vi "Control and acquisition.vi"() -> ()   [LabVIEW 2017]
uses:
  <vilib>/vision/Image Controls.llb/IMAQ Image.ctl
  <vilib>/vision/driver/IMAQdx.llb/IMAQdx Buffer Number Mode.ctl
  <vilib>/Utility/error.llb/DialogType.ctl
  <vilib>/vision/driver/IMAQdx.llb/IMAQdx Acquisition Mode.ctl
  <vilib>/DAQmx/write.llb/DAQmx Write (Analog 1D DBL NChan 1Samp).vi
  <vilib>/DAQmx/write.llb/DAQmx Write (Analog 1D Wfm NChan NSamp).vi
  <vilib>/DAQmx/create/channels.llb/DAQmx Create Channel (CO-Pulse Generation-Time).vi
  <vilib>/DAQmx/configure/timing.llb/DAQmx Timing (Implicit).vi
  <vilib>/vision/driver/Vision Acquisition Express Utility VIs.llb/Vision Acquisition Path Convert (Path).vi
  <vilib>/DAQmx/create/channels.llb/DAQmx Create Channel (AO-Voltage-Basic).vi
  <vilib>/DAQmx/miscellaneous.llb/DAQmx Fill In Error Info.vi
  <vilib>/DAQmx/configure/timing.llb/DAQmx Timing (Use Waveform).vi
  <vilib>/DAQmx/configure/trigger.llb/DAQmx Start Trigger (Digital Edge).vi
  <vilib>/vision/driver/NI_Vision_Acquisition_Software.lvlib
  <resource>/objmgr/imaqdx.rc
  <resource>/objmgr/daqmx.rc
  <vilib>/vision/NI_Vision_Development_Module.lvlib
panel:
  in  "?":dbl=40.0 format="%.1f"
  in  "Center laser\nfor power\nmeasurements":bool
  in  "Duration (ms)":dbl=10.5
  out "Multipoint":bool
  out "How to use:":string
  in  "Select mode:":u16(ring) items=["Line stimulation", "Hexagon shape stimulation"]
  out "FAST number of buffers":u32
  out "WIDE number of buffers":u32
  in  "?":dbl=2.0 format="%#_2f"
  in  "?":u32=500
  in  "?":dbl=2.0 format="%.1f"
  in  "Jump size (cm)":dbl=0.03791
  out "XY Graph":cluster{dbl[], dbl[]}(graph)
  out "(M)ULTI":bool
  in  "timeout (s)":dbl=10.0 format="%0.2f"
  in  "stop (T)":bool=TRUE
  in  "error in":errorcluster
  out "error out 2":errorcluster caption="error out"
  out "task out":refnum<k21>
  out "Time of previous recording":timestamp
  out "Trigger camera":bool
  in  "Initial Delay (ms)":dbl=0.5 caption="Initial delay (s)" format="%#.1f"
  in  "Pulse duration":dbl=0.003 caption="Pulse duration (ms)" format="%#.1p"
  in  "Number of pulses":i32=10
  in  "Interpulse interval":dbl=0.097 format="%#.1p"
  out "Boolean":bool
  out "LostBufferCount":u32
  out "new picture":picture
  in  "error in 3":errorcluster caption="error in"
  out "Image Out 2":T1(plugin-control)
  out "All Image Buffers Out 2":T1[](array[typedef])
  out "error out 3":errorcluster
  in  "Stop (F) 2":bool caption="Stop (F)"
  out "?":dbl format="%1_2f"
  out "Recording 2":bool
  out "Wide":bool
  in  "error in 2":errorcluster caption="error in"
  out "All Image Buffers Out":T1[](array[typedef])
  out "error out":errorcluster
  in  "Stop (F)":bool
  out "Frame Rate":dbl
  out "BufferCount":u32
  out "Recording":bool
  out "Fast":bool
  in  "color(black)":u32(colorbox)=6618880
  out "Xsaved1":dbl format="%#_2g"
  out "Ysaved1":dbl format="%#_2g"
  out "Ysaved2":dbl format="%#_2g"
  out "Xsaved2":dbl format="%#_2g"
  out "'1'":bool
  out "'2'":bool
  out "X":dbl format="%#_3f"
  out "Y":dbl format="%#_3f"
  out "Image Out":T1(plugin-control)
  out "x .and. y?":bool
  # "Cameras"
  # "Wide"
  # "Fast"
  # "FPS"
  # "Length (s)"
  # "Re-run VI to change these settings"
  # "Pulse generator"
  # "Re-run VI to change these settings"
  # "Patterned stimulation \nmode"
  # "Monitoring"
  # "System ready?"
  # "Stimulation shape:"
  # "Cameras?"
  # "Galvos?"
  # "Laser?"
  # "ON"
  # "FPS"
  # "FPS"
  # "rec?"
  # "rec?"
  # "Patterns?"
  # "ON"
types:
  T1 = typedef "IMAQ Image.ctl" = refnum<image>
  T2 = cluster{"Width":u16, "Style":enum32{"Solid", "Dash", "Dot", "DashDot", "DashDotDot"}}
  T3 = typedef "LVPoint32TypeDef.ctl" = cluster{"Horizontal":i32, "Vertical":i32}
  T4 = typedef "DialogType.ctl" = u16
  T5 = typedef "NI_Vision_Acquisition_Software.lvlib/IMAQdx Buffer Number Mode.ctl" = enum32{"Next", "Last", "Buffer Number", "Every", "Last New"}
  T6 = typedef "NI_Vision_Acquisition_Software.lvlib/IMAQdx Acquisition Mode.ctl" = enum32{"One Shot", "Continuous"}
  T7 = typedef "IMAQdx.ctl" = refnum<k21>
  T8 = cluster{"File Type":string, "Quality":u32, "Compress":bool, "Lossless":bool, "Ratio":sgl, "Codec":string, "Frame Rate":u32, "Limit Frames":bool, "FAST number of buffers":u32}
  T9 = cluster{"File Type":string, "Quality":u32, "Compress":bool, "Lossless":bool, "Ratio":sgl, "Codec":string, "Frame Rate":u32, "Limit Frames":bool, "WIDE number of buffers":u32}
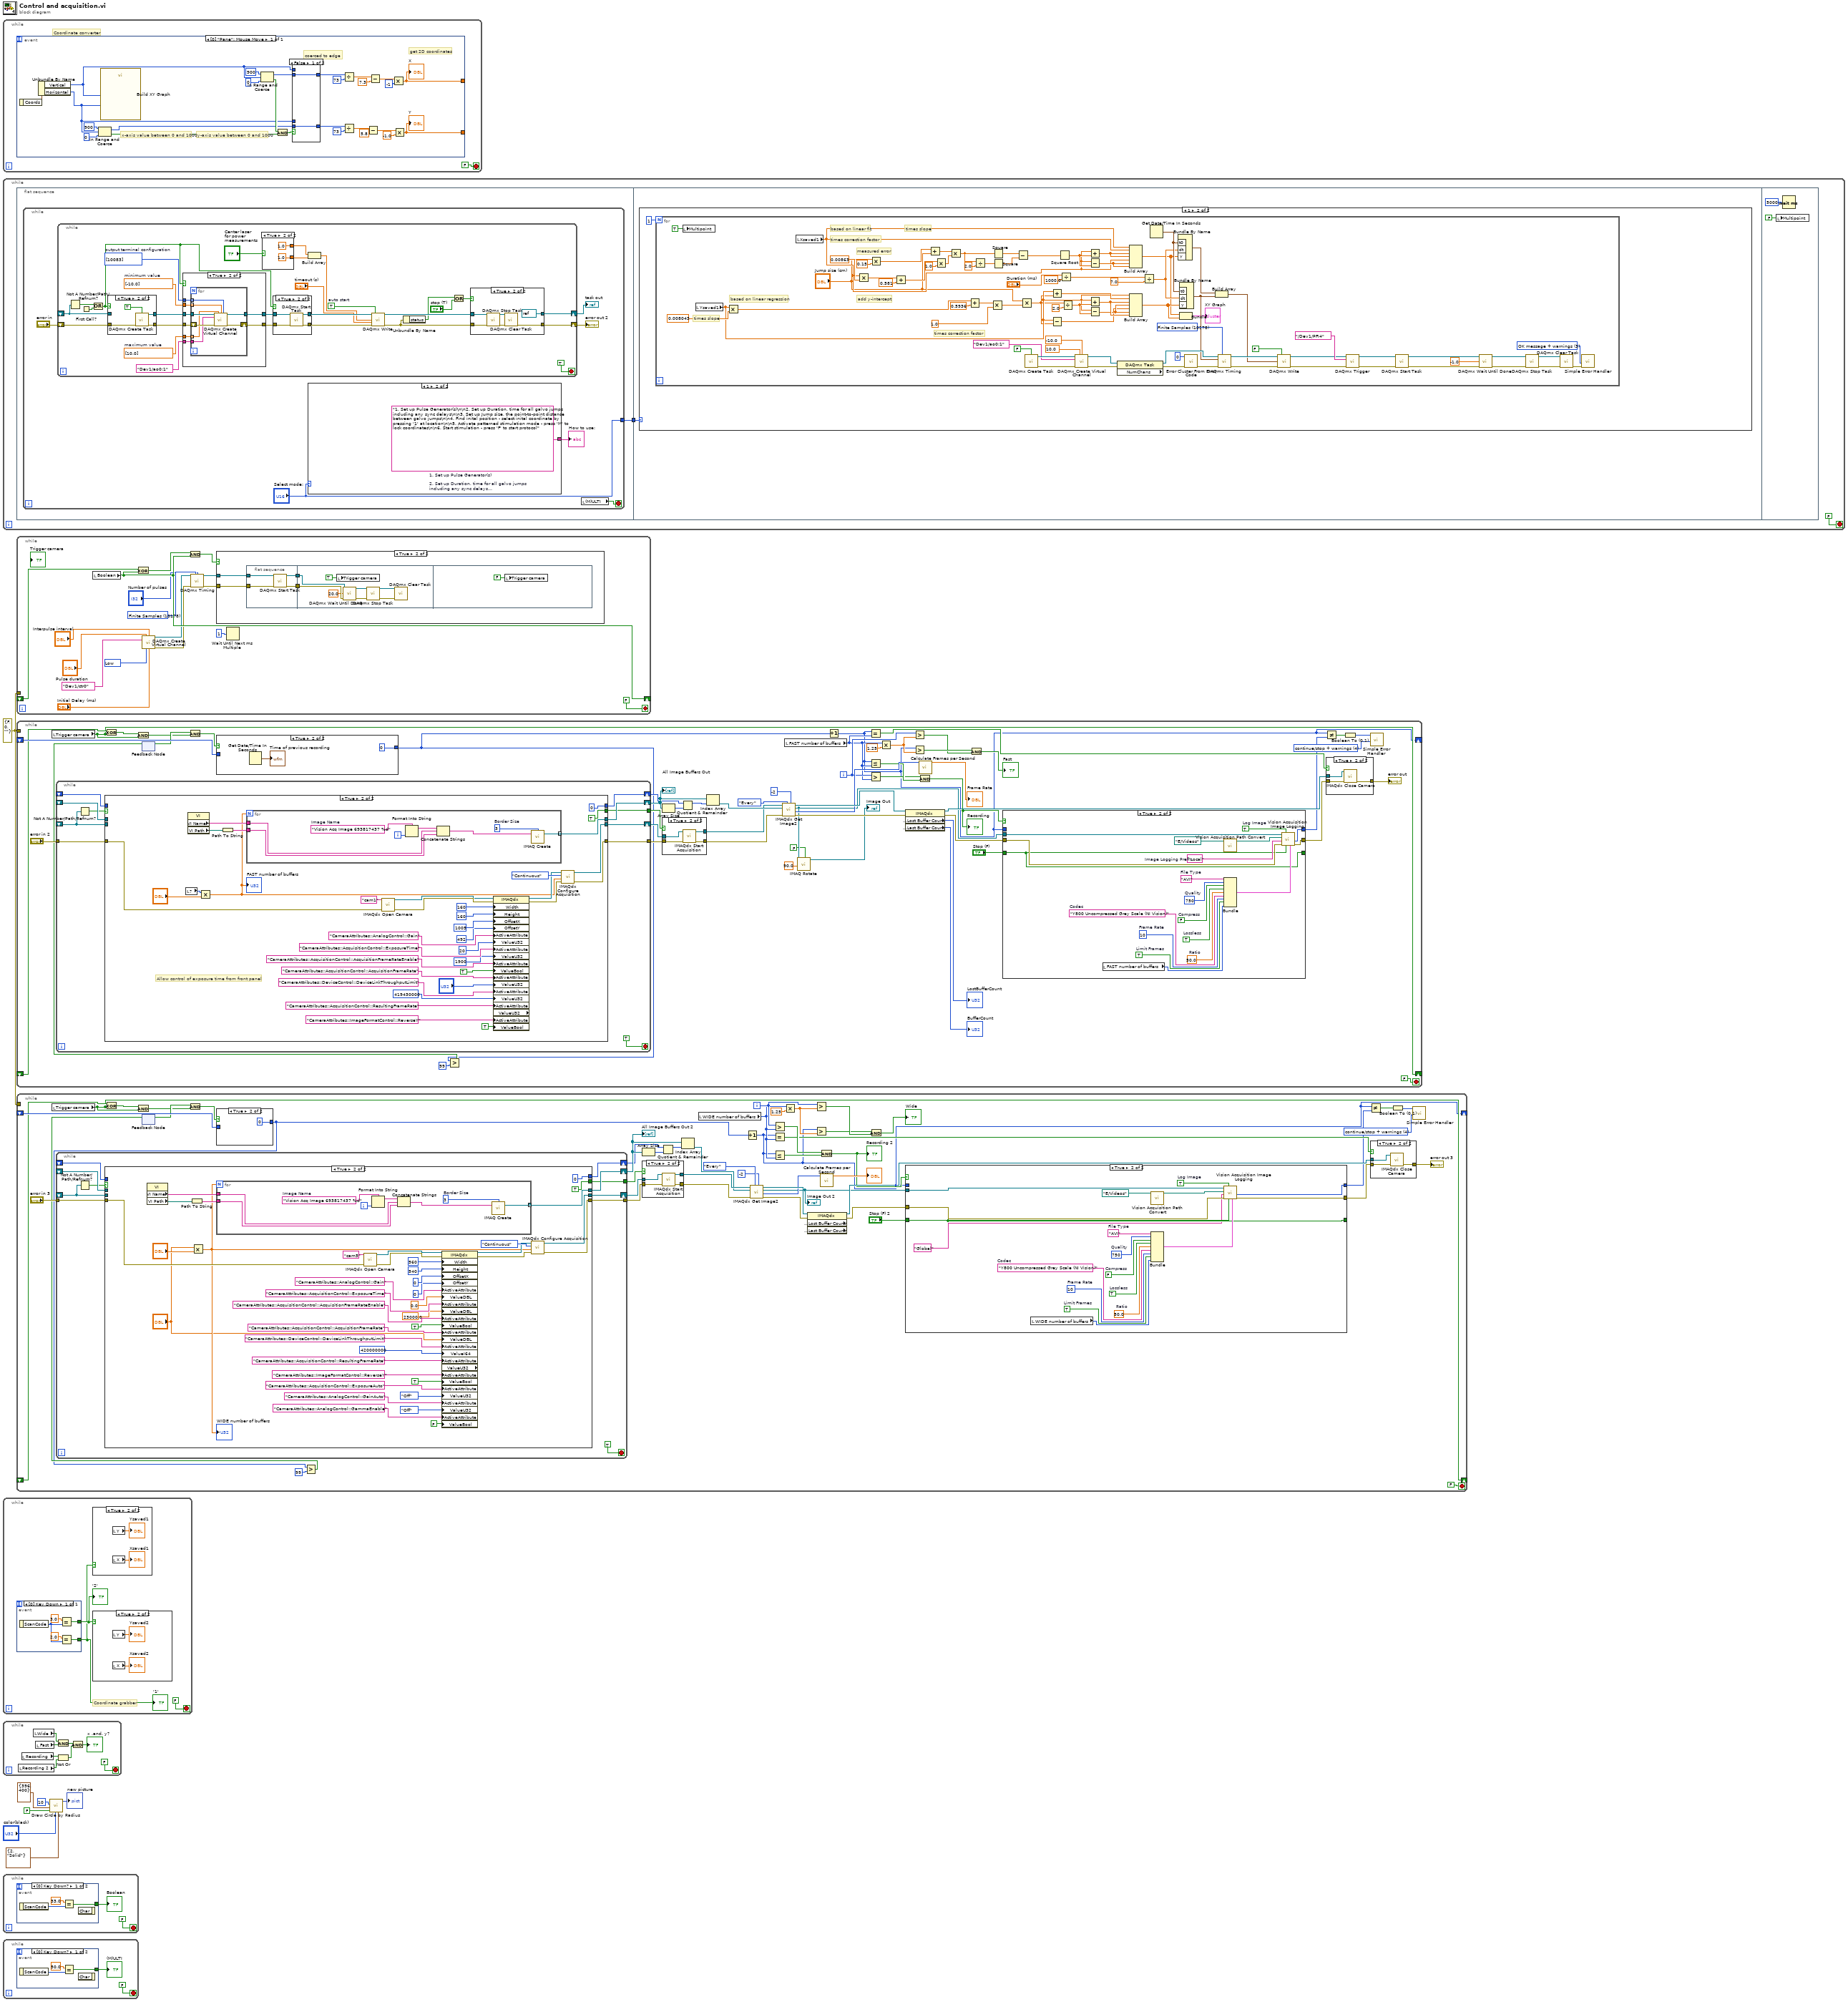
[diagram p0: block diagram]
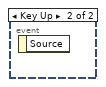
[diagram p2: hidden frame]
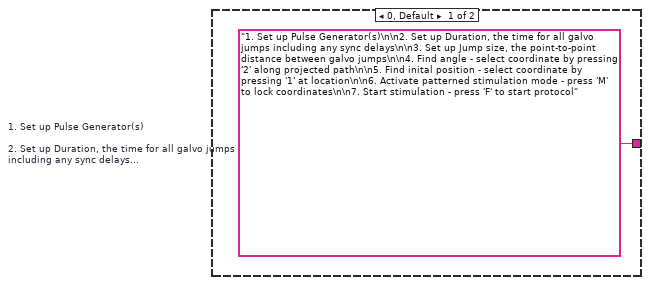
[diagram p3: hidden frame]
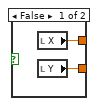
[diagram p4: hidden frame]
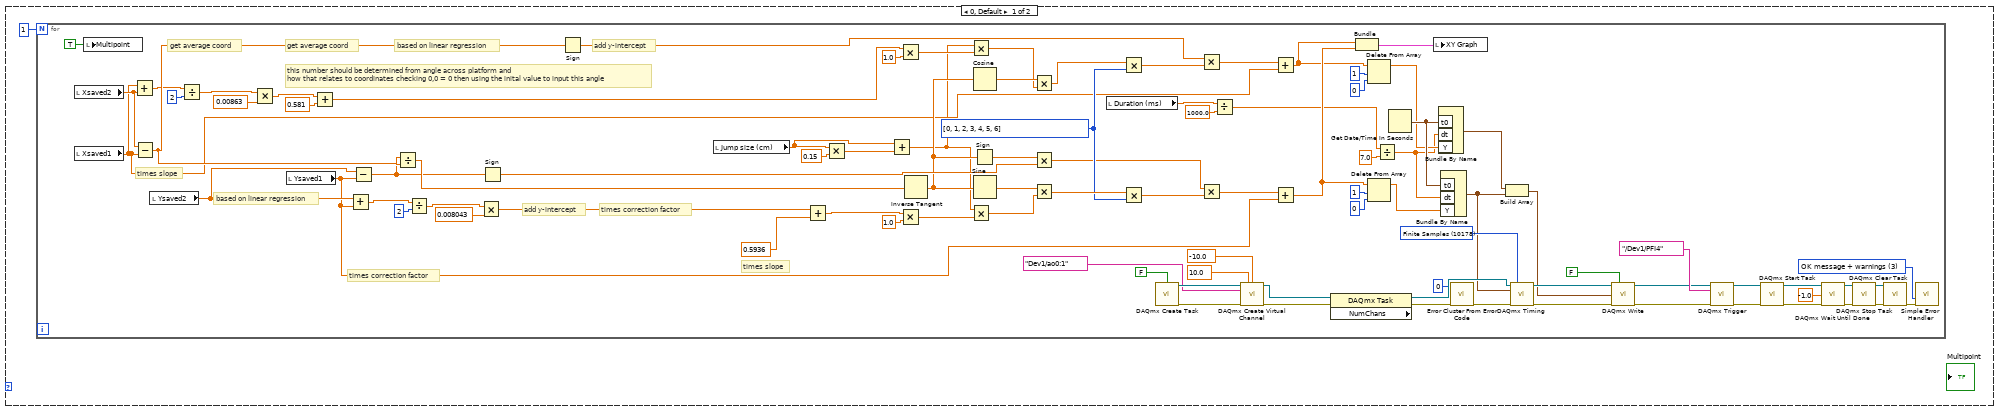
[diagram p9: hidden frame]
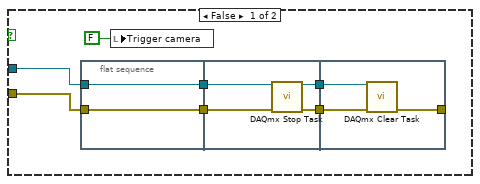
[diagram p10: hidden frame]
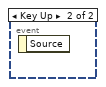
[diagram p11: hidden frame]
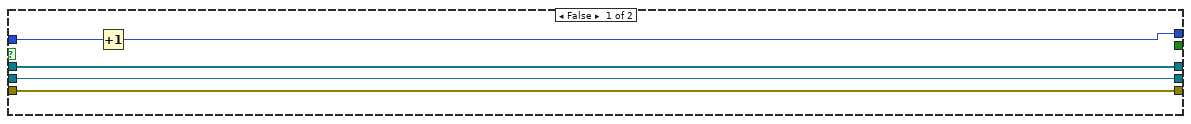
[diagram p16: hidden frame]
diagram:
  w1 = errorcluster {"status"=FALSE, "code"=0, "source"=""} ("error constant")
  n1 = while {
    stop <- FALSE ("stop") stop-if-true
    # "Coordinate converter"
    n2 = event shown="[0] \"Pane\": Mouse Move" {
      selector: _ -> [_]
      dyn-events: _ -> [_]
      timeout: _ -> [_]
      tunnel: [w14] -> _
      tunnel: [w12] -> _
      event Mouse Move {
        # "coerced to edge"
        # "y-axis value between 0 and 1000"
        # "x-axis value between 0 and 1000"
        # "get 2D coordinates"
        n3 = event-data() -> ("Coords"=w15:T3)  [unwired: 1 in]
        n4 = Unbundle By Name(w15) -> ("Vertical"=w10:i32, "Horizontal"=w9:i32)
        n5 = In Range and Coerce(upper limit=900, x=w9, lower limit=0) -> (coerced(x)=w22:i32, In Range?=w30:bool)
        n6 = call "Build XY Graph"("Y Input"=w9, "X Input"=w10) -> ()  [unwired: 8 in, 2 out]
        n7 = In Range and Coerce(upper limit=900, x=w10, lower limit=0) -> (coerced(x)=w23:i32, In Range?=w29:bool)
        n8 = And(x=w29, y=w30) -> (x .and. y?=w26:bool)
        n9 = case shown="False" w26 {
          tunnel: [w36 w38] -> w25
          tunnel: w10 -> [_ w38]
          tunnel: w9 -> [_ w37]
          tunnel: [w35 w37] -> w24
          tunnel: w23 -> [w36 _]
          tunnel: w22 -> [w35 _]
          frame False {
          }
          frame True {
          }
        }
        n10 = Divide(x=w25, y=73) -> (x/y=w17:dbl)
        n11 = Divide(x=w24, y=73) -> (x/y=w19:dbl)
        n12 = Subtract(x=w19, y=5.8) -> (x-y=w13:dbl)
        n13 = Subtract(x=w17, y=7.3) -> (x-y=w16:dbl)
        n14 = Multiply(x=w16, y=-1) -> (x*y=w14:dbl)
        "X" <- w14
        n15 = Multiply(x=w13, y=-1.0) -> (x*y=w12:dbl)
        "Y" <- w12
      }
    }
  }
  n16 = while {
    stop <- FALSE stop-if-true
    n17 = flat-sequence {
      tunnel: [w41] -> w39
      tunnel: w39 -> [w121]
      frame #0 {
        n18 = while {
          tunnel: ["Select mode:"] -> w41
          stop <- w44 stop-if-true
          n19 = while {
            shift-right: [w61] -> w45
            shift-left: _ -> [w75]
            shift-right: [w59] -> w46
            shift-left: "error in" -> [w76]
            stop <- TRUE stop-if-true
            w63 = TRUE  # auto start
            w69 = i32[] [10083] items=["Default"=-1, "RSE"=10083, "Differential"=10106, "Pseudodifferential"=12529]  # output terminal configuration
            w70 = dbl[] [10.0]  # maximum value
            w71 = dbl[] [-10.0]  # minimum value
            n20 = Not A Number/Path/Refnum?(number/path/refnum=w75) -> (NaN/Path/Refnum?=w74:bool)
            n21 = First Call?() -> (First Call?: T/F=w77:bool)
            n22 = Or(x=w74, y=w77) -> (x .or. y?=w68:bool)
            n23 = case shown="True" w68 {
              tunnel: [w116 w120] -> w73
              tunnel: w75 -> [w116 _]
              tunnel: [w115 w119] -> w72
              tunnel: w76 -> [w115 w117]
              frame False {
              }
              frame True {
                n24 = call <vilib>:"DAQmx Create Task.vi"("auto cleanup"=TRUE, "error in"=w117) -> ("task out"=w120:refnum<k21>, "error out"=w119:errorcluster)  [unwired: 12 in]
              }
            }
            n25 = case shown="True" w68 {
              tunnel: [w98 w104] -> w67
              tunnel: w73 -> [w98 w106]
              tunnel: [w97 w103] -> w66
              tunnel: w72 -> [w97 w105]
              tunnel: w71 -> [_ w102]
              tunnel: w70 -> [_ w101]
              tunnel: w69 -> [_ w100]
              tunnel: tag "Dev1/ao0:1" ("Physical Channel") -> [_ w99]
              frame False {
              }
              frame True {
                n26 = for {
                  tunnel: w106 -> [w114]
                  tunnel: [w112] -> w104
                  tunnel: w102 -> [w110] mode=indexing
                  tunnel: w101 -> [w109] mode=indexing
                  shift-right: [w111] -> w103
                  shift-left: w105 -> [w113]
                  tunnel: w100 -> [w108] mode=indexing
                  tunnel: w99 -> [w107]
                  n27 = call-poly <vilib>:"DAQmx Create Virtual Channel.vi"("task in"=w114, "maximum value"=w109, "minimum value"=w110, "output terminal configuration"=w108, "physical channels"=w107, "error in"=w113) -> ("task out"=w112:refnum<k21>, "error out"=w111:errorcluster)  [unwired: 8 in]
                }
              }
            }
            n28 = case shown="True" "Center laser\nfor power\nmeasurements" {
              tunnel: [w80 1.0 ("X")] -> w52
              tunnel: [w79 1.0 ("Y")] -> w51
              frame False {
                n29 = local read "X"() -> (w80:dbl)
                n30 = local read "Y"() -> (w79:dbl)
              }
              frame True {
              }
            }
            n31 = case shown="True" w68 {
              tunnel: [w92 w95] -> w65
              tunnel: w67 -> [w92 w96]
              tunnel: [w91 w93] -> w64
              tunnel: w66 -> [w91 w94]
              frame False {
              }
              frame True {
                n32 = call <vilib>:"DAQmx Start Task.vi"("task/channels in"=w96, "error in"=w94) -> ("task out"=w95:refnum<k21>, "error out"=w93:errorcluster)  [unwired: 12 in]
              }
            }
            n33 = Build Array(w52, w51) -> (w53:dbl[])
            n34 = call-poly <vilib>:"DAQmx Write.vi"("task/channels in"=w65, "auto start"=w63, "data"=w53, "timeout"="timeout (s)", "error in"=w64) -> ("task out"=w60:refnum<k21>, "error out"=w58:errorcluster)  [unwired: 8 in, 1 out]
            n35 = Unbundle By Name(w58) -> ("status"=w57:bool)
            n36 = Or(x=w57, y="stop (T)") -> (x .or. y?=w55:bool)
            n37 = case shown="True" w55 {
              tunnel: [w84 refnum<k21> refnum ("task in")] -> w61
              tunnel: w60 -> [w84 w90]
              tunnel: [w83 w87] -> w59
              tunnel: w58 -> [w83 w89]
              frame False {
              }
              frame True {
                n38 = call <vilib>:"DAQmx Stop Task.vi"("task/channels in"=w90, "error in"=w89) -> ("task out"=w86:refnum<k21>, "error out"=w88:errorcluster)  [unwired: 12 in]
                n39 = call <vilib>:"DAQmx Clear Task.vi"("task in"=w86, "error in"=w88) -> ("error out"=w87:errorcluster)  [unwired: 13 in]
              }
            }
          }
          "error out 2" <- w46
          "task out" <- w45
          n40 = case shown="1" "Select mode:" {
            tunnel: [w48 w49] -> w43
            frame 0, Default {
              w48 = "1. Set up Pulse Generator(s)\n\n2. Set up Duration, the time for all galvo jumps including any sync delays\n\n3. Set up Jump size, the point-to-point distance between galvo jumps\n\n4. Find angle - select coordinate by pressing '2' along projected path\n\n5. Find inital position - select coordinate by pressing '1' at location\n\n6. Activate patterned stimulation mode - press 'M' to lock coordinates\n\n7. Start stimulation - press 'F' to start protocol"  # 1. Set up Pulse Generator(s)  2. Set up Duration, the time for all galvo jumps including any sync delays  3. Set up Jump size, the point-to-point distance between galvo jumps  4. Find angle - select coordinate by pressing '2' along projected path  5. Find inital position - select coordinate by pressing '1' at location  6. Activate patterned stimulation mode - press 'M' to lock coordinates  7. Start stimulation - press 'F' to start protocol
            }
            frame 1 {
              w49 = "1. Set up Pulse Generator(s)\n\n2. Set up Duration, time for all galvo jumps including any sync delays\n\n3. Set up Jump size, the point-to-point distance between galvo jumps\n\n4. Find inital position - select inital coordinate by pressing '1' at location\n\n5. Activate patterned stimulation mode - press 'M' to lock coordinates\n\n6. Start stimulation - press 'F' to start protocol"  # 1. Set up Pulse Generator(s)  2. Set up Duration, time for all galvo jumps including any sync delays  3. Set up Jump size, the point-to-point distance between galvo jumps  4. Find inital position - select inital coordinate by pressing '1' at location  5. Activate patterned stimulation mode - press 'M' to lock coordinates  6. Start stimulation - press 'F' to start protocol
            }
          }
          "How to use:" <- w43
          n41 = local read "(M)ULTI"() -> (w44:bool)
        }
      }
      frame #1 {
        n42 = case shown="1" w121 {
          frame 0, Default {
            n43 = for {
              N: 1 -> [_]
              w154 = i32[] [0, 1, 2, 3, 4, 5, 6]
              w200 = 10178 items=["Finite Samples"=10178, "Continuous Samples"=10123] ("sample mode")
              w210 = T4 3 items=["no dialog", "OK message", "continue or stop message", "OK message + warnings", "continue/stop + warnings"] ("type of dialog (OK msg:1)")
              # "times correction factor"
              # "add y-intercept"
              # "times slope"
              # "get average coord"
              # "based on linear regression"
              # "times correction factor"
              # "add y-intercept"
              # "times slope"
              # "get average coord"
              # "based on linear regression"
              # "this number should be determined from angle across platform and \nhow that relates to coordinates checking 0,0 = 0 then using the inital value to input this angle"
              n44 = local read "Xsaved2"() -> (w161:dbl)
              n45 = local read "Xsaved1"() -> (w132:dbl)
              n46 = local write "Multipoint"(TRUE ("Multipoint")) -> ()
              n47 = Add(x=w132, y=w161) -> (x+y=w179:dbl)
              n48 = Subtract(x=w161, y=w132) -> (x-y=w184:dbl)
              n49 = local read "Ysaved2"() -> (w160:dbl)
              n50 = Divide(x=w179, y=2) -> (x/y=w177:dbl)
              n51 = Multiply(x=w177, y=0.00863) -> (x*y=w175:dbl)
              n52 = local read "Ysaved1"() -> (w142:dbl)
              n53 = Add(x=w175, y=0.581) -> (x+y=w173:dbl)
              n54 = Add(x=w160, y=w142) -> (x+y=w170:dbl)
              n55 = Subtract(x=w160, y=w142) -> (x-y=w183:dbl)
              n56 = Divide(x=w183, y=w184) -> (x/y=w190:dbl)
              n57 = Divide(x=w170, y=2) -> (x/y=w168:dbl)
              n58 = Multiply(x=w168, y=0.008043) -> (x*y=w166:dbl)
              n59 = Sign(1:w183) -> (0:w140:dbl)
              n60 = Sign(1:w184) -> (0:w143:dbl)
              n61 = local read "Jump size (cm)"() -> (w129:dbl)
              n62 = Add(x=w166, y=0.5936) -> (x+y=w164:dbl)
              n63 = Multiply(x=w129, y=0.15) -> (x*y=w130:dbl)
              n64 = Add(x=w129, y=w130) -> (x+y=w123:dbl)
              n65 = Multiply(x=w173, y=1.0) -> (x*y=w171:dbl)
              n66 = Multiply(x=w164, y=1.0) -> (x*y=w162:dbl)
              n67 = Inverse Tangent(1:w190) -> (0:w139:dbl)
              n68 = Multiply(x=w123, y=w171) -> (x*y=w138:dbl)
              n69 = Multiply(x=w123, y=w162) -> (x*y=w141:dbl)
              n70 = Cosine(x=w139) -> (cos(x)=w157:dbl)
              n71 = Sign(1:w139) -> (0:w149:dbl)
              n72 = Sine(x=w139) -> (sin(x)=w155:dbl)
              n73 = Multiply(x=w157, y=w138) -> (x*y=w158:dbl)
              n74 = Multiply(x=w149, y=w140) -> (x*y=w148:dbl)
              n75 = Multiply(x=w155, y=w141) -> (x*y=w156:dbl)
              n76 = local read "Duration (ms)"() -> (w133:dbl)
              n77 = Multiply(x=w158, y=w154) -> (x*y=w150:dbl[])
              n78 = Multiply(x=w156, y=w154) -> (x*y=w152:dbl[])
              n79 = call <vilib>:"DAQmx Create Task.vi"("auto cleanup"=FALSE) -> ("task out"=w203:refnum<k21>, "error out"=w204:errorcluster)  [unwired: 13 in]
              n80 = Multiply(x=w143, y=w150) -> (x*y=w151:dbl[])
              n81 = Multiply(x=w148, y=w152) -> (x*y=w153:dbl[])
              n82 = Divide(x=w133, y=1000.0) -> (x/y=w126:dbl)
              n83 = call-poly <vilib>:"DAQmx Create Virtual Channel.vi"("task in"=w203, "maximum value"=10.0 ("Maximum Value"), "minimum value"=-10.0 ("Minimum Value"), "physical channels"=tag "Dev1/ao0:1" ("Physical Channel"), "error in"=w204) -> ("task out"=w214:refnum<k21>, "error out"=w212:errorcluster)  [unwired: 9 in]
              n84 = Add(x=w151, y=w132) -> (x+y=w134:dbl[])
              n85 = Add(x=w153, y=w142) -> (x+y=w135:dbl[])
              n86 = property class="DAQmx Task" props=["NumChans"](reference=w214, error in=w212) -> (reference out=w206:refnum<k21>, error out=w213:errorcluster)  [unwired: 1 out]
              n87 = Bundle(w134, w135) -> (w159:cluster{dbl[], dbl[]})  [unwired: 1 in]
              n88 = Delete From Array(array=w134, length=1, index=0) -> (array with subset deleted=w136:dbl[])  [unwired: 1 out]
              n89 = Delete From Array(array=w135, length=1, index=0) -> (array with subset deleted=w137:dbl[])  [unwired: 1 out]
              n90 = Divide(x=w126, y=7.0) -> (x/y=w124:dbl)
              n91 = Get Date/Time In Seconds() -> (seconds since 1Jan1904=w199:timestamp)
              n92 = local write "XY Graph"(w159) -> ()
              n93 = Bundle By Name("t0"=w199, "dt"=w124, "Y"=w136) -> (w181:waveform(dbl))  [unwired: 1 in]
              n94 = Bundle By Name("t0"=w199, "dt"=w124, "Y"=w137) -> (w180:waveform(dbl))  [unwired: 1 in]
              n95 = call <vilib>:"Error Cluster From Error Code.vi"("error in (no error)"=w213, "error code (0)"=0) -> ("error out"=w197:errorcluster)  [unwired: 7 in]
              n96 = Build Array(w181, w180) -> (w189:waveform(dbl)[])
              n97 = call-poly <vilib>:"DAQmx Timing.vi"("task/channels in"=w206, "sample mode"=w200, "waveform"=w180, "error in"=w197) -> ("task out"=w202:refnum<k21>, "error out"=w198:errorcluster)  [unwired: 10 in]
              n98 = call-poly <vilib>:"DAQmx Write.vi"("task/channels in"=w202, "auto start"=FALSE, "data"=w189, "error in"=w198) -> ("task out"=w187:refnum<k21>, "error out"=w186:errorcluster)  [unwired: 9 in, 1 out]
              n99 = call-poly <vilib>:"DAQmx Trigger.vi"("task/channels in"=w187, "source"=tag "/Dev1/PFI4", "error in"=w186) -> ("task out"=w127:refnum<k21>, "error out"=w128:errorcluster)  [unwired: 11 in]
              n100 = call <vilib>:"DAQmx Start Task.vi"("task/channels in"=w127, "error in"=w128) -> ("task out"=w208:refnum<k21>, "error out"=w207:errorcluster)  [unwired: 12 in]
              n101 = call <vilib>:"DAQmx Wait Until Done.vi"("task/channels in"=w208, "timeout (sec)"=-1.0, "error in"=w207) -> ("task out"=w195:refnum<k21>, "error out"=w194:errorcluster)  [unwired: 11 in]
              n102 = call <vilib>:"DAQmx Stop Task.vi"("task/channels in"=w195, "error in"=w194) -> ("task out"=w192:refnum<k21>, "error out"=w193:errorcluster)  [unwired: 12 in]
              n103 = call <vilib>:"DAQmx Clear Task.vi"("task in"=w192, "error in"=w193) -> ("error out"=w209:errorcluster)  [unwired: 13 in]
              n104 = call <vilib>:"Simple Error Handler.vi"("type of dialog (OK msg:1)"=w210, "error in (no error)"=w209) -> ()  [unwired: 3 in, 5 out]
            }
          }
          frame 1 {
            n105 = for {
              N: 1 -> [_]
              w278 = 10178 items=["Finite Samples"=10178, "Continuous Samples"=10123] ("sample mode")
              w288 = T4 3 items=["no dialog", "OK message", "continue or stop message", "OK message + warnings", "continue/stop + warnings"] ("type of dialog (OK msg:1)")
              # "measured error"
              # "times correction factor"
              # "add y-intercept"
              # "times slope"
              # "based on linear regression"
              # "times correction factor"
              # "add y-intercept"
              # "times slope"
              # "based on linear fit"
              n106 = local write "Multipoint"(TRUE ("Multipoint")) -> ()
              n107 = local read "Ysaved1"() -> (w235:dbl)
              n108 = Multiply(x=w235, y=0.008043) -> (x*y=w254:dbl)
              n109 = local read "Xsaved1"() -> (w224:dbl)
              n110 = Multiply(x=w224, y=0.00863) -> (x*y=w260:dbl)
              n111 = Multiply(x="Jump size (cm)", y=0.15) -> (x*y=w222:dbl)
              n112 = Add(x=w260, y=0.581) -> (x+y=w258:dbl)
              n113 = Add(x=w222, y="Jump size (cm)") -> (x+y=w227:dbl)
              n114 = Multiply(x=w258, y=1.0) -> (x*y=w256:dbl)
              n115 = Multiply(x=w227, y=w256) -> (x*y=w233:dbl)
              n116 = Add(x=w254, y=0.5936) -> (x+y=w252:dbl)
              n117 = Divide(x=w233, y=2.0 ("x")) -> (x/y=w238:dbl)
              n118 = Multiply(x=w252, y=1.0) -> (x*y=w250:dbl)
              n119 = Square(x=w233) -> (x^2=w248:dbl)
              n120 = Square(x=w238) -> (x^2=w247:dbl)
              n121 = Subtract(x=w248, y=w247) -> (x-y=w246:dbl)
              n122 = Multiply(x="Jump size (cm)", y=w250) -> (x*y=w234:dbl)
              n123 = call <vilib>:"DAQmx Create Task.vi"("auto cleanup"=FALSE) -> ("task out"=w281:refnum<k21>, "error out"=w282:errorcluster)  [unwired: 13 in]
              n124 = Add(x=w235, y=w234) -> (x+y=w243:dbl)
              n125 = Subtract(x=w235, y=w234) -> (x-y=w239:dbl)
              n126 = Square Root(x=w246) -> (sqrt(x)=w240:dbl)
              n127 = Divide(x="Duration (ms)", y=1000.0) -> (x/y=w230:dbl)
              n128 = Divide(x=w234, y=2.0) -> (x/y=w236:dbl)
              n129 = call-poly <vilib>:"DAQmx Create Virtual Channel.vi"("task in"=w281, "maximum value"=10.0 ("Maximum Value"), "minimum value"=-10.0 ("Minimum Value"), "physical channels"=tag "Dev1/ao0:1" ("Physical Channel"), "error in"=w282) -> ("task out"=w292:refnum<k21>, "error out"=w290:errorcluster)  [unwired: 9 in]
              n130 = Add(x=w224, y=w240) -> (x+y=w245:dbl)
              n131 = Subtract(x=w224, y=w240) -> (x-y=w242:dbl)
              n132 = Add(x=w235, y=w236) -> (x+y=w244:dbl)
              n133 = Subtract(x=w235, y=w236) -> (x-y=w241:dbl)
              n134 = property class="DAQmx Task" props=["NumChans"](reference=w292, error in=w290) -> (reference out=w284:refnum<k21>, error out=w291:errorcluster)  [unwired: 1 out]
              n135 = Build Array(w224, w224, w245, w245, w224, w242, w242) -> (w228:dbl[])
              n136 = Build Array(w235, w243, w244, w241, w239, w241, w244) -> (w232:dbl[])
              n137 = Divide(x=w230, y=7.0) -> (x/y=w229:dbl)
              n138 = Get Date/Time In Seconds() -> (seconds since 1Jan1904=w277:timestamp)
              n139 = Bundle By Name("t0"=w277, "dt"=w229, "Y"=w228) -> (w263:waveform(dbl))  [unwired: 1 in]
              n140 = Bundle By Name("t0"=w277, "dt"=w229, "Y"=w232) -> (w262:waveform(dbl))  [unwired: 1 in]
              n141 = Bundle(w228, w232) -> (→"XY Graph":cluster{dbl[], dbl[]})  [unwired: 1 in]
              n142 = call <vilib>:"Error Cluster From Error Code.vi"("error in (no error)"=w291, "error code (0)"=0) -> ("error out"=w275:errorcluster)  [unwired: 7 in]
              n143 = Build Array(w263, w262) -> (w268:waveform(dbl)[])
              n144 = call-poly <vilib>:"DAQmx Timing.vi"("task/channels in"=w284, "sample mode"=w278, "waveform"=w262, "error in"=w275) -> ("task out"=w280:refnum<k21>, "error out"=w276:errorcluster)  [unwired: 10 in]
              n145 = call-poly <vilib>:"DAQmx Write.vi"("task/channels in"=w280, "auto start"=FALSE, "data"=w268, "error in"=w276) -> ("task out"=w266:refnum<k21>, "error out"=w265:errorcluster)  [unwired: 9 in, 1 out]
              n146 = call-poly <vilib>:"DAQmx Trigger.vi"("task/channels in"=w266, "source"=tag "/Dev1/PFI4", "error in"=w265) -> ("task out"=w226:refnum<k21>, "error out"=w225:errorcluster)  [unwired: 11 in]
              n147 = call <vilib>:"DAQmx Start Task.vi"("task/channels in"=w226, "error in"=w225) -> ("task out"=w286:refnum<k21>, "error out"=w285:errorcluster)  [unwired: 12 in]
              n148 = call <vilib>:"DAQmx Wait Until Done.vi"("task/channels in"=w286, "timeout (sec)"=-1.0, "error in"=w285) -> ("task out"=w273:refnum<k21>, "error out"=w272:errorcluster)  [unwired: 11 in]
              n149 = call <vilib>:"DAQmx Stop Task.vi"("task/channels in"=w273, "error in"=w272) -> ("task out"=w270:refnum<k21>, "error out"=w271:errorcluster)  [unwired: 12 in]
              n150 = call <vilib>:"DAQmx Clear Task.vi"("task in"=w270, "error in"=w271) -> ("error out"=w287:errorcluster)  [unwired: 13 in]
              n151 = call <vilib>:"Simple Error Handler.vi"("type of dialog (OK msg:1)"=w288, "error in (no error)"=w287) -> ()  [unwired: 3 in, 5 out]
            }
          }
        }
      }
      frame #2 {
        n152 = local write "Multipoint"(FALSE ("Multipoint")) -> ()
        n153 = Wait (ms)(milliseconds to wait=u32 5000) -> ()  [unwired: 1 out]
      }
    }
  }
  n154 = while {
    stop <- FALSE stop-if-true
    # "Coordinate grabber"
    n155 = event shown="[0] Key Down" {
      selector: _ -> [_]
      dyn-events: _ -> [_]
      timeout: _ -> [_]
      tunnel: [w306] -> w298
      tunnel: [w305] -> w299
      event Key Down {
        n156 = event-data() -> ("ScanCode"=w304:i16)  [unwired: 1 in]
        n157 = Equal?(x=3.0, y=w304) -> (x = y?=w305:bool)
        n158 = Equal?(x=2.0, y=w304) -> (x = y?=w306:bool)
      }
    }
    "'2'" <- w299
    "'1'" <- w298
    n159 = case shown="True" w298 {
      frame False {
      }
      frame True {
        n160 = local read "Y"() -> (→"Ysaved1":dbl)
        n161 = local read "X"() -> (→"Xsaved1":dbl)
      }
    }
    n162 = case shown="True" w299 {
      frame False {
      }
      frame True {
        n163 = local read "Y"() -> (→"Ysaved2":dbl)
        n164 = local read "X"() -> (→"Xsaved2":dbl)
      }
    }
  }
  n165 = while {
    stop <- FALSE stop-if-true
    n166 = local read "Recording 2"() -> (w315:bool)
    n167 = local read "Recording"() -> (w316:bool)
    n168 = local read "Wide"() -> (w313:bool)
    n169 = local read "Fast"() -> (w312:bool)
    n170 = And(x=w313, y=w312) -> (x .and. y?=w311:bool)
    n171 = Not Or(1:w315, 2:w316) -> (0:w310:bool)
    n172 = And(x=w311, y=w310) -> (x .and. y?=→"x .and. y?":bool)
  }
  n173 = while {
    stop <- FALSE stop-if-true
    n174 = event shown="[0] Key Down?" {
      selector: _ -> [_ _]
      dyn-events: _ -> [_ _]
      timeout: _ -> [_ _]
      tunnel: [w320 _] -> w317
      event Key Down? {
        n175 = event-data() -> ("ScanCode"=w319:i16)  [unwired: 1 in]
        n176 = Equal?(x=33.0, y=w319) -> (x = y?=w320:bool)
        n177 = event-data() -> ()  [unwired: 2 in, 1 out]
      }
      event Key Up {
        n178 = event-data() -> ()  [unwired: 1 in, 1 out]
      }
    }
    "Boolean" <- w317
  }
  n179 = while {
    stop <- FALSE stop-if-true
    n180 = event shown="[0] Key Down?" {
      selector: _ -> [_ _]
      dyn-events: _ -> [_ _]
      timeout: _ -> [_ _]
      tunnel: [w324 _] -> w322
      event Key Down? {
        n181 = event-data() -> ("ScanCode"=w325:i16)  [unwired: 1 in]
        n182 = Equal?(x=50.0, y=w325) -> (x = y?=w324:bool)
        n183 = event-data() -> ()  [unwired: 2 in, 1 out]
      }
      event Key Up {
        n184 = event-data() -> ()  [unwired: 1 in, 1 out]
      }
    }
    "(M)ULTI" <- w322
  }
  n185 = while {
    shift-right: [w340] -> _
    shift-left: _ -> [w339]
    tunnel: w1 -> [_]
    stop <- FALSE ("stop 2") stop-if-true
    w334 = 10178 items=["Finite Samples"=10178, "Continuous Samples"=10123, "Hardware Timed Single Point"=12522] ("sample mode")
    w336 = 10214 items=["High"=10192, "Low"=10214] ("Idle State")
    n186 = local read "Boolean"() -> (w340:bool)
    n187 = Exclusive Or(1:w340, 2:w339) -> (0:w342:bool)
    n188 = call-poly <vilib>:"DAQmx Create Virtual Channel.vi"("high time"="Pulse duration", "low time"="Interpulse interval", "counter"=tag "Dev1/ctr0" ("Counter(s)"), "idle state"=w336, "initial delay"="Initial Delay (ms)") -> ("task out"=w335:refnum<k21>, "error out"=w333:errorcluster)  [unwired: 9 in]
    n189 = And(x=w342, y=w340) -> (x .and. y?=w341:bool)
    n190 = call-poly <vilib>:"DAQmx Timing.vi"("task/channels in"=w335, "sample mode"=w334, "samples per channel"="Number of pulses", "error in"=w333) -> ("task out"=w331:refnum<k21>, "error out"=w330:errorcluster)  [unwired: 10 in]
    n191 = case shown="True" w341 {
      tunnel: w330 -> [w349 w363]
      tunnel: w331 -> [w350 w362]
      frame False {
        n192 = flat-sequence {
          tunnel: w349 -> [w351]
          tunnel: w350 -> [w352]
          tunnel: [w352] -> w348
          tunnel: [w351] -> w347
          tunnel: w348 -> [w355]
          tunnel: w347 -> [w354]
          tunnel: [w356] -> w346
          tunnel: [w353] -> w345
          tunnel: [w358] -> _
          tunnel: w346 -> [w357]
          tunnel: w345 -> [w359]
          frame #0 {
          }
          frame #1 {
            n193 = call <vilib>:"DAQmx Stop Task.vi"("task/channels in"=w355, "error in"=w354) -> ("task out"=w356:refnum<k21>, "error out"=w353:errorcluster)  [unwired: 12 in]
          }
          frame #2 {
            n194 = call <vilib>:"DAQmx Clear Task.vi"("task in"=w357, "error in"=w359) -> ("error out"=w358:errorcluster)  [unwired: 13 in]
          }
        }
        n195 = local write "Trigger camera"(FALSE) -> ()
      }
      frame True {
        n196 = flat-sequence {
          tunnel: [w366] -> w361
          tunnel: [w367] -> w360
          tunnel: w362 -> [w365]
          tunnel: w363 -> [w364]
          tunnel: w360 -> [w375]
          tunnel: w361 -> [w374]
          frame #0 {
            n197 = call <vilib>:"DAQmx Start Task.vi"("task/channels in"=w365, "error in"=w364) -> ("task out"=w367:refnum<k21>, "error out"=w366:errorcluster)  [unwired: 12 in]
          }
          frame #1 {
            n198 = local write "Trigger camera"(TRUE) -> ()
            n199 = call <vilib>:"DAQmx Wait Until Done.vi"("task/channels in"=w375, "timeout (sec)"=20.0, "error in"=w374) -> ("task out"=w373:refnum<k21>, "error out"=w372:errorcluster)  [unwired: 11 in]
            n200 = call <vilib>:"DAQmx Stop Task.vi"("task/channels in"=w373, "error in"=w372) -> ("task out"=w371:refnum<k21>, "error out"=w370:errorcluster)  [unwired: 12 in]
            n201 = call <vilib>:"DAQmx Clear Task.vi"("task in"=w371, "error in"=w370) -> ()  [unwired: 13 in, 1 out]
          }
          frame #2 {
            n202 = local write "Trigger camera"(FALSE) -> ()
          }
        }
      }
    }
    n203 = Wait Until Next ms Multiple(millisecond multiple=u32 1) -> ()  [unwired: 1 out]
  }
  n204 = while {
    shift-right: [w386] -> _
    shift-left: _ -> [w402]
    shift-right: [w400] -> _
    shift-left: _ -> [w401]
    tunnel: w1 -> [_]
    i -> [w393]
    stop <- FALSE stop-if-true
    w381 = T4 4 items=["no dialog", "OK message", "continue or stop message", "OK message + warnings", "continue/stop + warnings"] ("type of dialog (OK msg:1)")
    n205 = local read "Trigger camera"() -> (w400:bool)
    n206 = while {
      shift-right: [w477] -> w422
      shift-left: _ -> [w469]
      tunnel: [w476] -> w430
      tunnel: "error in 2" -> [w475]
      shift-right: [w473] -> w426
      shift-left: _ -> [w472]
      shift-right: [w471] -> w419
      shift-left: _ -> [w470]
      tunnel: [w467] -> w418
      stop <- TRUE stop-if-true
      n207 = Not A Number/Path/Refnum?(number/path/refnum=w469) -> (NaN/Path/Refnum?=w468:bool)
      n208 = case shown="True" w468 {
        tunnel: [w482 w515] -> w477
        tunnel: w469 -> [w482 _]
        tunnel: [w481 w514] -> w476
        tunnel: w475 -> [w481 w517]
        tunnel: [w480 w513] -> w473
        tunnel: w472 -> [w480 _]
        tunnel: [w478 0] -> w471
        tunnel: w470 -> [w479 _]
        tunnel: [_ TRUE] -> w467
        frame False {
          n209 = Increment(x=w479) -> (x+1=w478:i32)
        }
        frame True {
          # "Allow control of exposure time from front panel"
          n210 = local read item#45() -> (w484:u32)
          n211 = property class="VI"() -> ("VI Name"=w510:string, "VI Path"=w511:path)  [unwired: 2 in, 2 out]
          n212 = Multiply(x=w484, y="?") -> (x*y=w485:dbl)
          "FAST number of buffers" <- w485
          n213 = Path To String(path=w511) -> (string=w509:string)
          n214 = for "For Loop_template0" {
            N: w485 -> [_]
            tunnel: [w525] -> w513 mode=indexing
            tunnel: w510 -> [w520]
            tunnel: w509 -> [w519]
            i -> [w524]
            w518 = 3  # Border Size
            w523 = "Vision Acq Image 693817437 %d"  # Image Name
            n215 = Format Into String(format string=w523, w524) -> (resulting string=w522:string)  [unwired: 2 in, 1 out]
            n216 = Concatenate Strings(w522, w520, w519) -> (w521:string)
            n217 = call "IMAQ Create"("Border Size"=w518, "Image Name"=w521) -> ("New Image"=w525:T1)  [unwired: 2 in, 2 out]
          }
          n218 = call <vilib>:"IMAQdx Open Camera.vi"("error in"=w517, "Session In"="cam1" ("Interface Name")) -> ("error out"=w494:errorcluster, "Session Out"=w493:T7)  [unwired: 1 in, 7 out]
          n219 = property class="IMAQdx" props=["Width", "Height", "OffsetX", "OffsetY", "ActiveAttribute", "ValueU32", "ActiveAttribute", "ValueU32", "ActiveAttribute", "ValueBool", "ActiveAttribute", "ValueU32", "ActiveAttribute", "ValueU32", "ActiveAttribute", "ValueU32", "ActiveAttribute", "ValueBool"](reference=w493, error in=w494, "Width"=u32 160 ("Height"), "Height"=u32 160 ("Width"), "OffsetX"=u32 1005, "OffsetY"=u32 492, "ActiveAttribute"="CameraAttributes::AnalogControl::Gain", "ValueU32"=u32 20, "ActiveAttribute"="CameraAttributes::AcquisitionControl::ExposureTime", "ValueU32"=u32 1900, "ActiveAttribute"="CameraAttributes::AcquisitionControl::AcquisitionFrameRateEnable", "ValueBool"=TRUE, "ActiveAttribute"="CameraAttributes::AcquisitionControl::AcquisitionFrameRate", "ValueU32"="?", "ActiveAttribute"="CameraAttributes::DeviceControl::DeviceLinkThroughputLimit", "ValueU32"=u32 419430000, "ActiveAttribute"="CameraAttributes::AcquisitionControl::ResultingFrameRate", "ActiveAttribute"="CameraAttributes::ImageFormatControl::ReverseY", "ValueBool"=TRUE) -> (reference out=w491:T7, error out=w492:errorcluster)  [unwired: 1 out]
          n220 = call <vilib>:"IMAQdx Configure Acquisition.vi"("error in"=w492, "Number of Buffers"=w485, "Continuous?"=IMAQdx_Acquisition_Mode."Continuous", "Session In"=w491) -> ("error out"=w514:errorcluster, "Session Out"=w515:T7)  [unwired: 6 out]
        }
      }
    }
    "All Image Buffers Out" <- w426
    n221 = Exclusive Or(1:w400, 2:w401) -> (0:w403:bool)
    n222 = And(x=w403, y=w400) -> (x .and. y?=w396:bool)
    n223 = feedback #1() -> (w397:bool)  [unwired: 1 in]
    n224 = And(x=w397, y=w396) -> (x .and. y?=w395:bool)
    n225 = case shown="True" w395 {
      tunnel: [w432 0] -> w394
      tunnel: w402 -> [w432 _]
      frame False {
      }
      frame True {
        n226 = Get Date/Time In Seconds() -> (seconds since 1Jan1904=→"Time of previous recording":timestamp)
      }
    }
    n227 = Greater?(x=w394, y=99) -> (0:w398:bool)
    n228 = feedback-in #1(w398) -> ()
    n229 = Array Size(array=w426) -> (size(s)=w427:i32)
    n230 = case shown="True" w418 {
      tunnel: w422 -> [w462 w466]
      tunnel: w430 -> [w461 w465]
      tunnel: [w461 w464] -> w420
      tunnel: [w462 w463] -> w421
      frame False {
      }
      frame True {
        n231 = call <vilib>:"IMAQdx Start Acquisition.vi"("error in"=w465, "Session In"=w466) -> ("error out"=w464:errorcluster, "Session Out"=w463:T7)  [unwired: 8 out]
      }
    }
    n232 = Quotient & Remainder(x=w419, y=w427) -> (x-y*floor(x/y)=w425:i32)  [unwired: 1 out]
    n233 = Index Array(array=w426, index=w425) -> (element=w424:T1)
    n234 = call <vilib>:"IMAQdx Get Image2.vi"("Timeout (ms)"=-2, "Buffer Number Mode (Next)"=IMAQdx_Buffer_Number_Mode."Every", "error in"=w420, "Image In"=w424, "Session In"=w421) -> ("error out"=w428:errorcluster, "Buffer Number Out"=w417:u32, "Image Out"=w379:T1, "Session Out"=w429:T7)  [unwired: 3 in]
    n235 = local read "FAST number of buffers"() -> (w390:u32)
    n236 = call "IMAQ Rotate"("Maintain Size"=FALSE, "Angle (degrees)"=sgl 90.0, "Image Src"=w379) -> ("Image Dst Out"=→"Image Out":T1)  [unwired: 7 in, 1 out]
    n237 = Increment(x=w394) -> (x+1=w386:i32)
    n238 = Equal?(x=w386, y=w390) -> (x = y?=w392:bool)
    n239 = Less Or Equal?(x=w386, y=w390) -> (x <= y?=w407:bool)
    n240 = Greater?(x=w393, y=w390) -> (0:w406:bool)
    n241 = Multiply(x=w390, y=1.25) -> (x*y=w387:dbl)
    n242 = property class="IMAQdx"(reference=w429, error in=w428) -> (reference out=w413:T7, error out=w423:errorcluster, "Status Information:Lost Buffer Count"=→"LostBufferCount":u32, "Status Information:Last Buffer Count"=→"BufferCount":u32)
    n243 = Greater?(x=w393, y=w387) -> (0:w384:bool)
    n244 = Greater?(x=w386, y=w387) -> (0:w385:bool)
    n245 = call <vilib>:"Calculate Frames per Second.vi"("Buffer Number"=w417) -> ("Acquired Frames/s"=→"Frame Rate":dbl)  [unwired: 2 in, 8 out]
    n246 = And(x=w406, y=w407) -> (x .and. y?=w405:bool)
    "Recording" <- w405
    n247 = And(x=w385, y=w384) -> (x .and. y?=→"Fast":bool)
    n248 = case shown="True" w405 {
      tunnel: w423 -> [w437 w456]
      tunnel: w379 -> [_ w439]
      tunnel: [w437 w442] -> w414
      tunnel: "Stop (F)" -> [w436 w443]
      tunnel: [w436 w443] -> _
      tunnel: [w435 w438] -> w389
      tunnel: w386 -> [w435 _]
      frame False {
      }
      frame True {
        w446 = TRUE  # Log Image
        w455 = "Local"  # Image Logging Prefix
        w450 = sgl 50.0  # Ratio
        w451 = TRUE  # Lossless
        w452 = FALSE  # Compress
        w453 = u32 750  # Quality
        w449 = "Y800 Uncompressed Grey Scale (NI Vision)"  # Codec
        w448 = u32 10  # Frame Rate
        w447 = TRUE  # Limit Frames
        w454 = "AVI"  # File Type
        n249 = local read "FAST number of buffers"() -> (w440:u32)
        n250 = call-poly <vilib>:"Vision Acquisition Path Convert.vi"("Path In"=path "E:/Videos") -> ("Path Out"=w444:path)  [unwired: 10 in]
        n251 = Bundle("File Type"=w454, "Quality"=w453, "Compress"=w452, "Lossless"=w451, "Ratio"=w450, "Codec"=w449, "Frame Rate"=w448, "Limit Frames"=w447, "FAST number of buffers"=w440) -> (w445:T8)  [unwired: 1 out]
        n252 = call <vilib>:"Vision Acquisition Image Logging.vi"("File Settings"=w445, "Close"=w443, "Log Image"=w446, "error in (no error)"=w456, "Image Logging Prefix"=w455, "Image Logging Path"=w444, "Image In"=w439) -> ("error out"=w442:errorcluster, "f"=w438:u32)  [unwired: 3 out]
      }
    }
    n253 = Not Equal?(x=w386, y=w389) -> (x != y?=w383:bool)
    n254 = case "Case Structure_template1" shown="True" w392 {
      tunnel: [w457 w459] -> w412
      tunnel: w414 -> [w457 w460]
      tunnel: w413 -> [_ w458]
      frame False {
      }
      frame True {
        n255 = call <vilib>:"IMAQdx Close Camera.vi"("error in"=w460, "Session In"=w458) -> ("error out"=w459:errorcluster)  [unwired: 9 out]
      }
    }
    "error out" <- w412
    n256 = Boolean To (0,1)(Boolean=w383) -> (0, 1=w382:i16)
    n257 = call <vilib>:"Simple Error Handler.vi"("error code (no error:0)"=w382, "type of dialog (OK msg:1)"=w381) -> ()  [unwired: 3 in, 5 out]
  }
  n258 = while {
    shift-right: [w531] -> _
    shift-left: _ -> [w553]
    shift-right: [w537] -> _
    shift-left: _ -> [w549]
    tunnel: w1 -> [_]
    i -> [w540]
    stop <- FALSE stop-if-true
    w530 = T4 4 items=["no dialog", "OK message", "continue or stop message", "OK message + warnings", "continue/stop + warnings"] ("type of dialog (OK msg:1)")
    n259 = local read "Trigger camera"() -> (w537:bool)
    n260 = while {
      shift-right: [w620] -> w567
      shift-left: _ -> [w612]
      tunnel: [w619] -> w574
      tunnel: "error in 3" -> [w618]
      shift-right: [w616] -> w570
      shift-left: _ -> [w615]
      shift-right: [w614] -> w564
      shift-left: _ -> [w613]
      tunnel: [w610] -> w563
      stop <- TRUE stop-if-true
      n261 = Not A Number/Path/Refnum?(number/path/refnum=w612) -> (NaN/Path/Refnum?=w611:bool)
      n262 = case shown="True" w611 {
        tunnel: [w625 w663] -> w620
        tunnel: w612 -> [w625 _]
        tunnel: [w624 w662] -> w619
        tunnel: w618 -> [w624 w665]
        tunnel: [w623 w661] -> w616
        tunnel: w615 -> [w623 _]
        tunnel: [w621 0] -> w614
        tunnel: w613 -> [w622 _]
        tunnel: [_ TRUE] -> w610
        frame False {
          n263 = Increment(x=w622) -> (x+1=w621:i32)
        }
        frame True {
          n264 = property class="VI"() -> ("VI Name"=w658:string, "VI Path"=w659:path)  [unwired: 2 in, 2 out]
          n265 = Path To String(path=w659) -> (string=w657:string)
          n266 = Multiply(x="?", y="?") -> (x*y=w638:dbl)
          "WIDE number of buffers" <- w638
          n267 = for "For Loop_template0" {
            N: w638 -> [_]
            tunnel: [w666] -> w661 mode=indexing
            tunnel: w658 -> [w669]
            tunnel: w657 -> [w668]
            i -> [w673]
            w667 = 3  # Border Size
            w672 = "Vision Acq Image 693817437 %d"  # Image Name
            n268 = Format Into String(format string=w672, w673) -> (resulting string=w671:string)  [unwired: 2 in, 1 out]
            n269 = Concatenate Strings(w671, w669, w668) -> (w670:string)
            n270 = call "IMAQ Create"("Border Size"=w667, "Image Name"=w670) -> ("New Image"=w666:T1)  [unwired: 2 in, 2 out]
          }
          n271 = call <vilib>:"IMAQdx Open Camera.vi"("error in"=w665, "Session In"="cam5" ("Interface Name")) -> ("error out"=w643:errorcluster, "Session Out"=w634:T7)  [unwired: 1 in, 7 out]
          n272 = property class="IMAQdx" props=["Width", "Height", "OffsetX", "OffsetY", "ActiveAttribute", "ValueDBL", "ActiveAttribute", "ValueDBL", "ActiveAttribute", "ValueBool", "ActiveAttribute", "ValueDBL", "ActiveAttribute", "ValueI64", "ActiveAttribute", "ValueU32", "ActiveAttribute", "ValueBool", "ActiveAttribute", "ValueU32", "ActiveAttribute", "ValueU32", "ActiveAttribute", "ValueBool"](reference=w634, error in=w643, "Width"=u32 560 ("Height"), "Height"=u32 540 ("Width"), "OffsetX"=u32 0, "OffsetY"=u32 0, "ActiveAttribute"="CameraAttributes::AnalogControl::Gain", "ValueDBL"=0.0, "ActiveAttribute"="CameraAttributes::AcquisitionControl::ExposureTime", "ValueDBL"=23000.0, "ActiveAttribute"="CameraAttributes::AcquisitionControl::AcquisitionFrameRateEnable", "ValueBool"=TRUE, "ActiveAttribute"="CameraAttributes::AcquisitionControl::AcquisitionFrameRate", "ValueDBL"="?", "ActiveAttribute"="CameraAttributes::DeviceControl::DeviceLinkThroughputLimit", "ValueI64"=i64 420000000, "ActiveAttribute"="CameraAttributes::AcquisitionControl::ResultingFrameRate", "ActiveAttribute"="CameraAttributes::ImageFormatControl::ReverseY", "ValueBool"=TRUE, "ActiveAttribute"="CameraAttributes::AcquisitionControl::ExposureAuto", "ValueU32"=enum16{"Off"}."Off", "ActiveAttribute"="CameraAttributes::AnalogControl::GainAuto", "ValueU32"=enum16{"Off"}."Off", "ActiveAttribute"="CameraAttributes::AnalogControl::GammaEnable", "ValueBool"=FALSE) -> (reference out=w641:T7, error out=w642:errorcluster)  [unwired: 1 out]
          n273 = call <vilib>:"IMAQdx Configure Acquisition.vi"("error in"=w642, "Number of Buffers"=w638, "Continuous?"=IMAQdx_Acquisition_Mode."Continuous", "Session In"=w641) -> ("error out"=w662:errorcluster, "Session Out"=w663:T7)  [unwired: 6 out]
        }
      }
    }
    "All Image Buffers Out 2" <- w570
    n274 = Exclusive Or(1:w537, 2:w549) -> (0:w548:bool)
    n275 = And(x=w548, y=w537) -> (x .and. y?=w544:bool)
    n276 = feedback #2() -> (w545:bool)  [unwired: 1 in]
    n277 = And(x=w545, y=w544) -> (x .and. y?=w543:bool)
    n278 = case shown="True" w543 {
      tunnel: [w576 0] -> w542
      tunnel: w553 -> [w576 _]
      frame False {
      }
      frame True {
      }
    }
    n279 = Greater?(x=w542, y=99) -> (0:w546:bool)
    n280 = feedback-in #2(w546) -> ()
    n281 = Array Size(array=w570) -> (size(s)=w571:i32)
    n282 = case shown="True" w563 {
      tunnel: w567 -> [w605 w609]
      tunnel: w574 -> [w604 w608]
      tunnel: [w604 w607] -> w565
      tunnel: [w605 w606] -> w566
      frame False {
      }
      frame True {
        n283 = call <vilib>:"IMAQdx Start Acquisition.vi"("error in"=w608, "Session In"=w609) -> ("error out"=w607:errorcluster, "Session Out"=w606:T7)  [unwired: 8 out]
      }
    }
    n284 = Quotient & Remainder(x=w564, y=w571) -> (x-y*floor(x/y)=w569:i32)  [unwired: 1 out]
    n285 = Index Array(array=w570, index=w569) -> (element=w527:T1)
    n286 = local read "WIDE number of buffers"() -> (w538:u32)
    n287 = Increment(x=w542) -> (x+1=w531:i32)
    n288 = call <vilib>:"IMAQdx Get Image2.vi"("Timeout (ms)"=-2, "Buffer Number Mode (Next)"=IMAQdx_Buffer_Number_Mode."Every", "error in"=w565, "Image In"=w527, "Session In"=w566) -> ("error out"=w572:errorcluster, "Buffer Number Out"=w562:u32, "Image Out"=w526:T1, "Session Out"=w573:T7)  [unwired: 3 in]
    "Image Out 2" <- w526
    n289 = Greater?(x=w540, y=w538) -> (0:w551:bool)
    n290 = Equal?(x=w531, y=w538) -> (x = y?=w541:bool)
    n291 = Less Or Equal?(x=w531, y=w538) -> (x <= y?=w552:bool)
    n292 = Multiply(x=w538, y=1.25) -> (x*y=w532:dbl)
    n293 = property class="IMAQdx" props=["Status Information:Lost Buffer Count", "Status Information:Last Buffer Count"](reference=w573, error in=w572) -> (reference out=w558:T7, error out=w568:errorcluster)  [unwired: 2 out]
    n294 = Greater?(x=w540, y=w532) -> (0:w534:bool)
    n295 = Greater?(x=w531, y=w532) -> (0:w533:bool)
    n296 = And(x=w551, y=w552) -> (x .and. y?=w550:bool)
    "Recording 2" <- w550
    n297 = call <vilib>:"Calculate Frames per Second.vi"("Buffer Number"=w562) -> ("Acquired Frames/s"=→"?":dbl)  [unwired: 2 in, 8 out]
    n298 = And(x=w533, y=w534) -> (x .and. y?=→"Wide":bool)
    n299 = case shown="True" w550 {
      tunnel: w568 -> [w580 w599]
      tunnel: w526 -> [_ w598]
      tunnel: [w580 w585] -> w559
      tunnel: "Stop (F) 2" -> [w579 w586]
      tunnel: [w579 w586] -> _
      tunnel: [w578 w582] -> w536
      tunnel: w531 -> [w578 _]
      frame False {
      }
      frame True {
        w589 = TRUE  # Log Image
        w593 = sgl 50.0  # Ratio
        w594 = TRUE  # Lossless
        w595 = FALSE  # Compress
        w596 = u32 750  # Quality
        w592 = "Y800 Uncompressed Grey Scale (NI Vision)"  # Codec
        w591 = u32 10  # Frame Rate
        w590 = TRUE  # Limit Frames
        w597 = "AVI"  # File Type
        n300 = local read "WIDE number of buffers"() -> (w583:u32)
        n301 = call-poly <vilib>:"Vision Acquisition Path Convert.vi"("Path In"=path "E:/Videos") -> ("Path Out"=w587:path)  [unwired: 10 in]
        n302 = Bundle("File Type"=w597, "Quality"=w596, "Compress"=w595, "Lossless"=w594, "Ratio"=w593, "Codec"=w592, "Frame Rate"=w591, "Limit Frames"=w590, "WIDE number of buffers"=w583) -> (w588:T9)  [unwired: 1 out]
        n303 = call <vilib>:"Vision Acquisition Image Logging.vi"("File Settings"=w588, "Close"=w586, "Log Image"=w589, "error in (no error)"=w599, "Image Logging Prefix"="Global" ("Mouse name"), "Image Logging Path"=w587, "Image In"=w598) -> ("error out"=w585:errorcluster, "f"=w582:u32)  [unwired: 3 out]
      }
    }
    n304 = Not Equal?(x=w531, y=w536) -> (x != y?=w529:bool)
    n305 = case "Case Structure_template1" shown="True" w541 {
      tunnel: [w600 w602] -> w557
      tunnel: w559 -> [w600 w603]
      tunnel: w558 -> [_ w601]
      frame False {
      }
      frame True {
        n306 = call <vilib>:"IMAQdx Close Camera.vi"("error in"=w603, "Session In"=w601) -> ("error out"=w602:errorcluster)  [unwired: 9 out]
      }
    }
    "error out 3" <- w557
    n307 = Boolean To (0,1)(Boolean=w529) -> (0, 1=w528:i16)
    n308 = call <vilib>:"Simple Error Handler.vi"("error code (no error:0)"=w528, "type of dialog (OK msg:1)"=w530) -> ()  [unwired: 3 in, 5 out]
  }
  n309 = call <vilib>:"Draw Circle by Radius.vi"("pen"=T2 {"Width"=2, "Style"=enum."Solid"}, "color(black)"="color(black)", "fill?(F)"=FALSE, "pixel center"=cluster{"horizontal":i16, "vertical":i16} {"horizontal"=396, "vertical"=400}, "radius"=i16 10) -> ("new picture"=→"new picture":picture)  [unwired: 6 in]
